vi "Do Read.vi"(8 "error in (no error)":errorcluster, 10 "Interface":refnum<class "Interface.lvclass">, 11 "Section 1 in":refnum<class "Section 1.lvclass">) -> (0 "error out":errorcluster, 2 "All Keys Found?":bool, 3 "Section 1 out":refnum<class "Section 1.lvclass">)   [LabVIEW 2013, in "LVOOP Introduction.lvlib" / "Section 1.lvclass"]
doc: "Read keys/value pairs from Interface.\n\nOverwriting dynamic dispatch VI."
uses:
  Section 1.lvclass
  Configuration/Classes/Interface/Interface.lvclass
  Configuration/Classes/Section/Section.lvclass
  Section 1.lvclass/Section 1.ctl
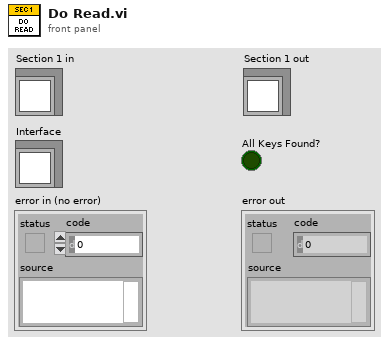
[diagram p1: front panel]
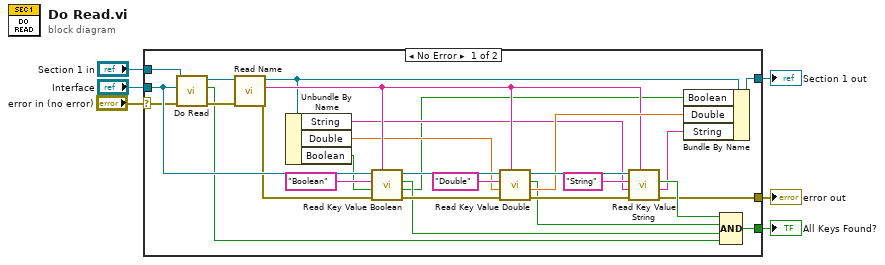
[diagram p0: block diagram]
diagram:
  n1 = case shown="No Error" "error in (no error)" {
    selector: "error in (no error)" -> [w7 w35]
    tunnel: "Section 1 in" -> [w34 w36]
    tunnel: [w33 w36] -> w5
    tunnel: "Interface" -> [w32 _]
    tunnel: [w13 w35] -> w3
    tunnel: [w11 _] -> w2
    frame No Error {
      n2 = call-parent "Do Read.vi"("error in (no error)"=w7, "Interface"=w32, "Section in"=w34) -> ("error out"=w26:errorcluster, "All Keys Found?"=w8:bool, "Section out"=w27:refnum<class "Section 1.lvclass">)  [unwired: 6 in]
      n3 = call "Read Name.vi"("error in (no error)"=w26, "Section in"=w27) -> ("error out"=w25:errorcluster, "Name"=w22:string, "Section out"=w19:refnum<class "Section 1.lvclass">)  [unwired: 7 in]
      n4 = Unbundle By Name(w19) -> ("String"=w16:string, "Double"=w17:dbl, "Boolean"=w18:bool)
      n5 = call-dynamic "Read Key Value Boolean.vi"("Section Name"=w22, "error in (no error)"=w25, "Default"=w18, "Key Name"="Boolean", "Interface in"=w32) -> ("error out"=w30:errorcluster, "Value"=w10:bool, "found"=w12:bool, "Interface out"=w31:refnum<class "Interface.lvclass">)  [unwired: 3 in]
      n6 = call-dynamic "Read Key Value Double.vi"("Section Name"=w22, "error in (no error)"=w30, "Default"=w17, "Key Name"="Double", "Interface in"=w31) -> ("error out"=w28:errorcluster, "Value"=w24:dbl, "found"=w14:bool, "Interface out"=w29:refnum<class "Interface.lvclass">)  [unwired: 3 in]
      n7 = call-dynamic "Read Key Value String.vi"("Section Name"=w22, "error in (no error)"=w28, "Default"=w16, "Key Name"="String", "Interface in"=w29) -> ("error out"=w13:errorcluster, "Value"=w9:string, "found"=w15:bool)  [unwired: 3 in, 1 out]
      n8 = Bundle By Name(cluster=w19, "Boolean"=w10, "Double"=w24, "String"=w9) -> (w33:refnum<class "Section 1.lvclass">)
      n9 = Compound Arithmetic op=AND(w15, w14, w12, w8) -> (w11:bool)
    }
    frame Error {
    }
  }
  "error out" <- w3
  "Section 1 out" <- w5
  "All Keys Found?" <- w2
